vi "Save Recall List Program.vi"(8 "error in (no error)":errorcluster, 9 "List Location (0)":u32 max=9 format="%#_0f", 10 "Save Recall List Program (0:Save)":u16(ring) items=["Save", "Recall"], 11 "VISA resource name":refnum<visa-resource-name>) -> (0 "error out":errorcluster, 3 "VISA resource name out":refnum<visa-resource-name>)   [LabVIEW 2018, in "BK Precision 983X Series.lvlib"]
doc: "Saves currently selected list program or recalls a list program.\n\nNote: If recalling a list and list parameters and list step parameters have not been saved yet, all information will be lost. Save the list first before performing a recall if a list is currently being edited."
uses:
  <instrlib>/BK Precision 983X Series/BK Precision 983X Series.lvlib
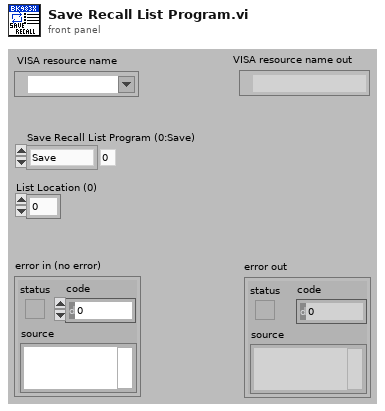
[diagram p1: front panel]
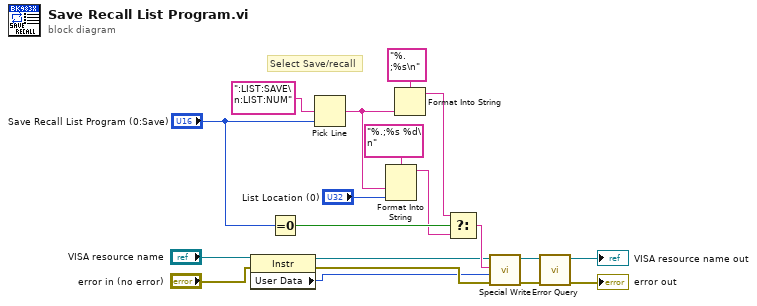
[diagram p0: block diagram]
diagram:
  # "Select Save/recall"
  n1 = property class="Instr"(reference="VISA resource name", error in="error in (no error)") -> (reference out=w4:refnum<visa-resource-name>, error out=w6:errorcluster, "User Data"=w5:u32)
  n2 = Equal To 0?(x="Save Recall List Program (0:Save)") -> (x = 0?=w14:bool)
  n3 = Pick Line(multi-line string=":LIST:SAVE\n:LIST:NUM", line index="Save Recall List Program (0:Save)") -> (output string=w3:string)  [unwired: 1 in]
  n4 = Format Into String(format string="%.;%s %d\n", w3, "List Location (0)") -> (resulting string=w13:string)  [unwired: 2 in, 1 out]
  n5 = Format Into String(format string="%.;%s\n", w3) -> (resulting string=w2:string)  [unwired: 2 in, 1 out]
  n6 = Select(t=w2, s=w14, f=w13) -> (s? t:f=w9:string)
  n7 = call <instrlib>:"Special Write.vi"("error in (no error)"=w6, "Delay (0 ms)"=w5, "Input String"=w9, "VISA resource name"=w4) -> ("error out"=w10:errorcluster, "VISA resource name out"=w11:refnum<visa-resource-name>)  [unwired: 6 in]
  n8 = call <instrlib>:"Error Query.vi"("error in (no error)"=w10, "VISA resource name"=w11) -> ("error out"=→"error out":errorcluster, "VISA resource name out"=→"VISA resource name out":refnum<visa-resource-name>)  [unwired: 6 in, 2 out]
